vi "CRYGraph Picture Window.vi"() -> ()   [LabVIEW 2013]
uses:
  Control/CRYPicture Property.ctl
  Control/CRYFlag Cluster.ctl
  SubVI/CRYData View Global.vi
  SubVI/CRYMain Sub Window Global.vi
  CRYCurveLibrary/Global/CRYCurve Library Global.vi
panel:
  in  "LoadFinish":bool
  out "Event Name":string
  in  "OpenProperty":bool
  out "PropertyTab":string
  out "Test":string
  in  "Cursor":string[][](table)
  out "Cursor Ref":refnum<vi>
  out "Queue Name":string
  in  "StateOut":bool
  in  "CursorShow":bool
  out "Picture Property":T1
  in  "Draw":bool
  out "Graph Ref":refnum<vi>
  out "Graph Number":i32
  in  "LegendShow":bool
  in  "stop":bool
  out "Legend Ref":refnum<vi>
  in  "Legend":i32(listbox) caption="Multicolumn Listbox"
  in  "GraphType":string
  out "Title Name":string
  out "GPicture":picture
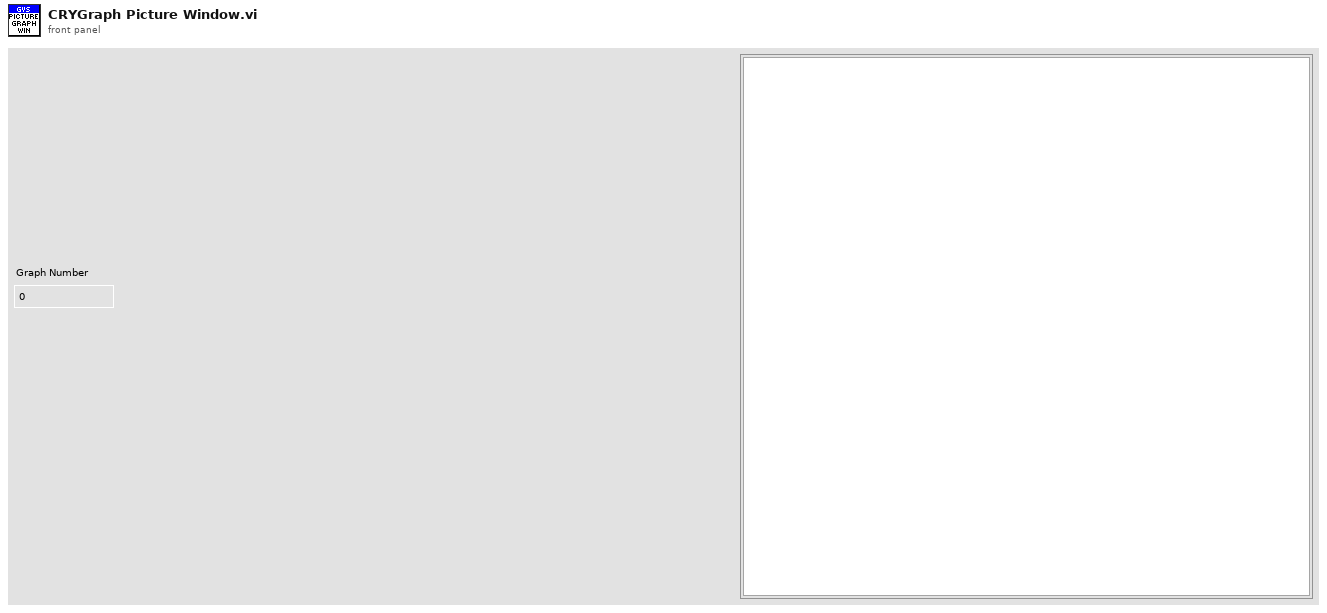
[diagram p1: front panel]
types:
  T1 = typedef "CRYPicture Property.ctl" = cluster{"Image Path":string, "Show vertical scroll bar":bool, "Show horizontal scroll bar":bool}
  T2 = typedef "CRYGraph Event.ctl" = cluster{"EvenName":string, "TitleName":string, "GraphName":string, "GraphType":string, "Data":variant, "Queue Name":string, "DataView Number":i32}
  T3 = typedef "CRYFlag Cluster.ctl" = cluster{"LegendShow":bool, "CellClick":bool, "Total Number":bool, "ScaleFitX":bool, "ScaleFitY":bool, "MapModeX":u8, "MapModeY":u8, "CursorShow":bool, "MagnitudeShow":bool, "PreviewShow":bool, "CursorEnabled":bool, "IntensityShow":bool, "PaletteShow":bool, "PhaseShow":bool, "XYShow":bool, "FrequencyShow":bool, "LegendVScrollShow":bool, "FrequencyVScrollShow":bool}
  T4 = enum16{"Left Button", "Center Button", "Right Button", "Window Close"}
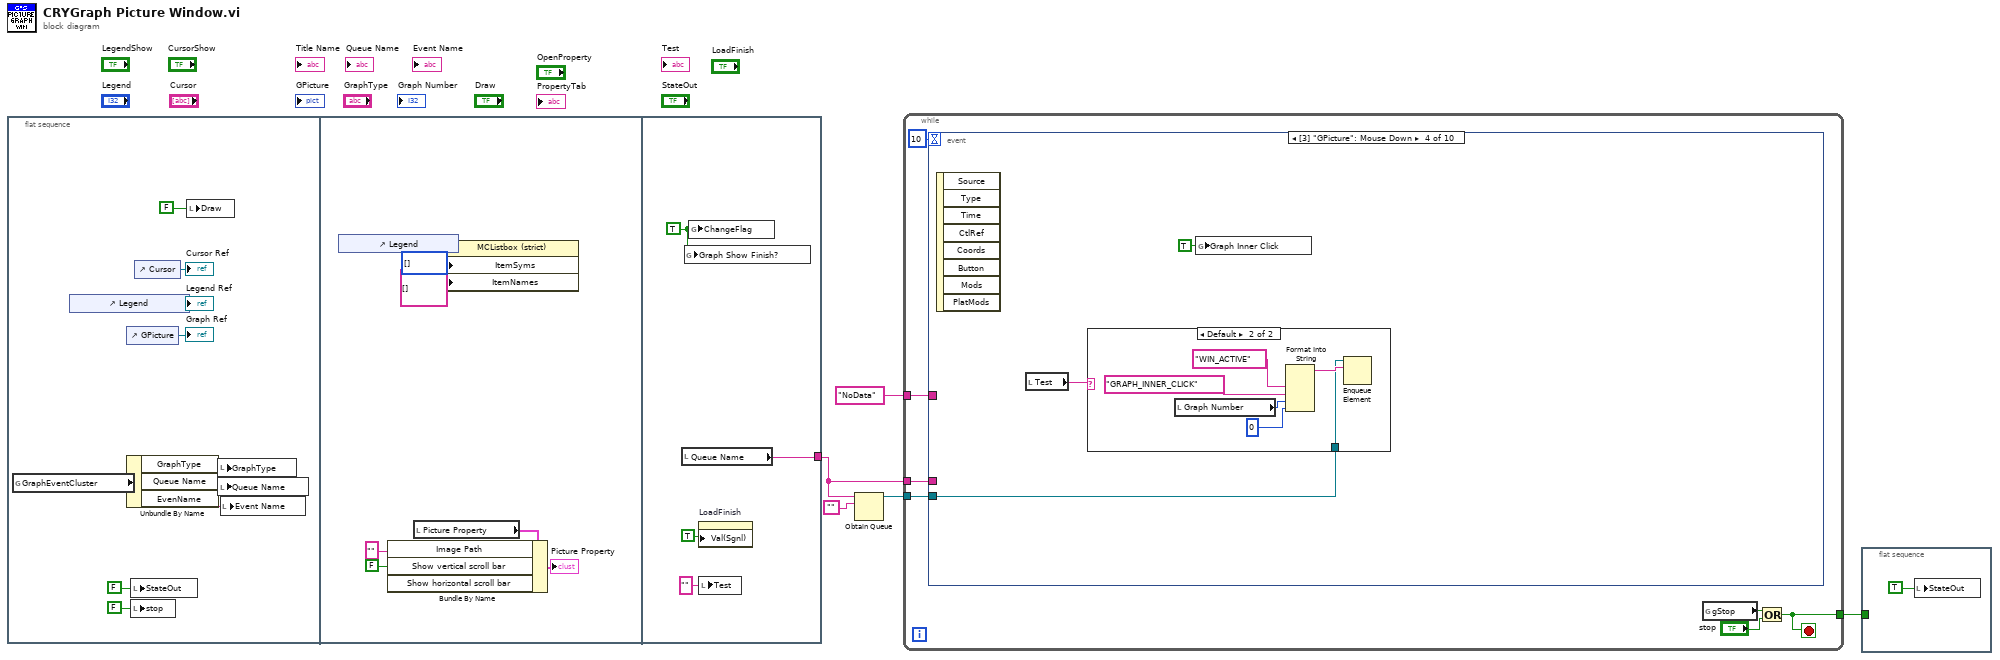
[diagram p0: block diagram]
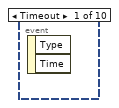
[diagram p2: hidden frame]
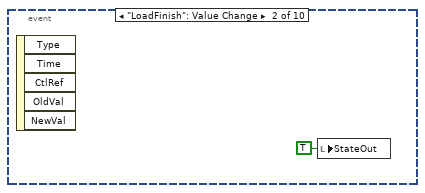
[diagram p3: hidden frame]
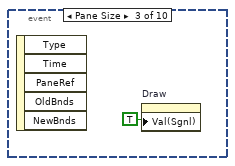
[diagram p4: hidden frame]
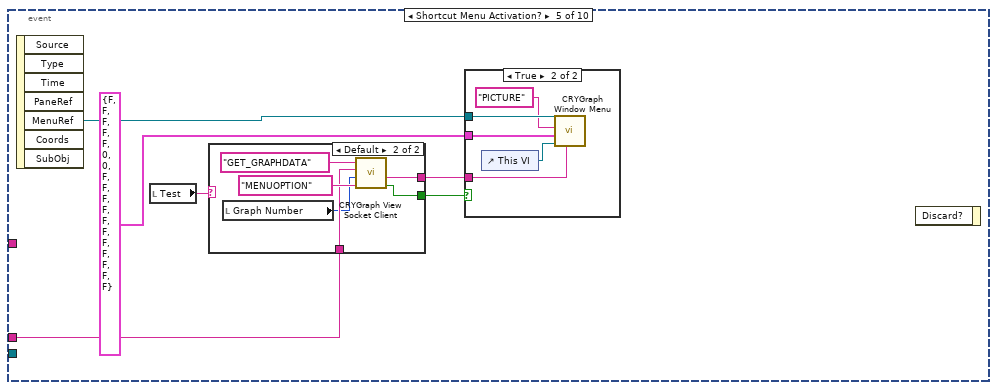
[diagram p6: hidden frame]
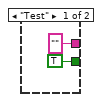
[diagram p7: hidden frame]
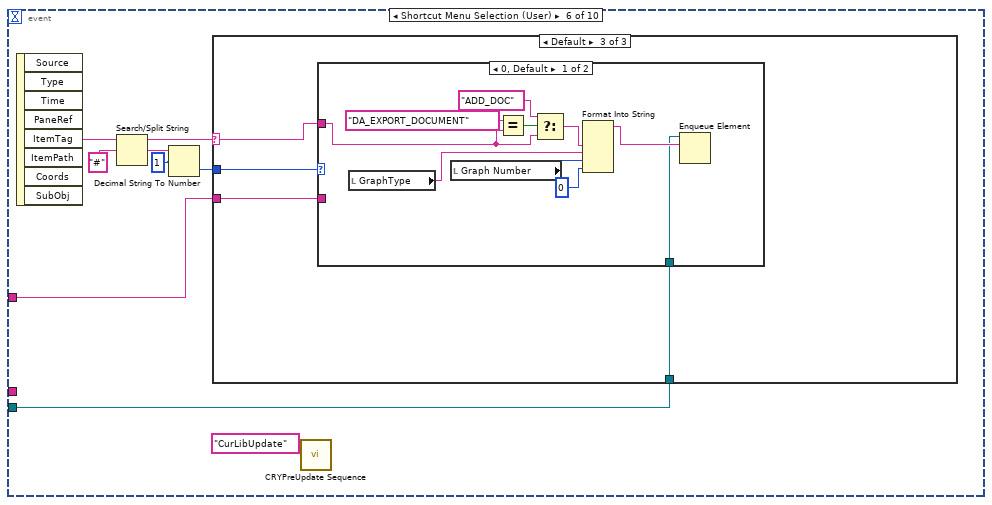
[diagram p9: hidden frame]
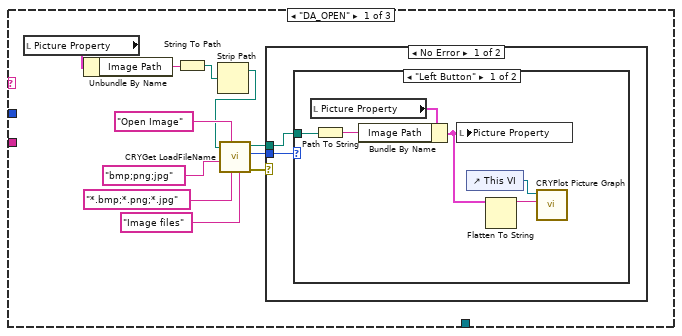
[diagram p10: hidden frame]
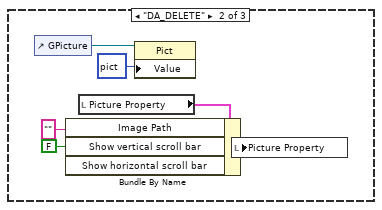
[diagram p13: hidden frame]
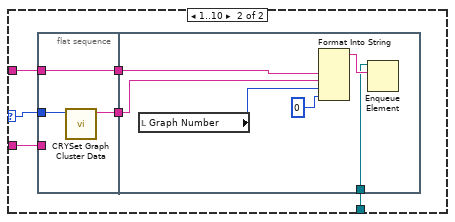
[diagram p14: hidden frame]
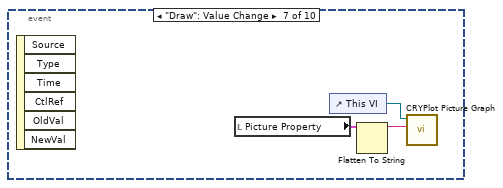
[diagram p15: hidden frame]
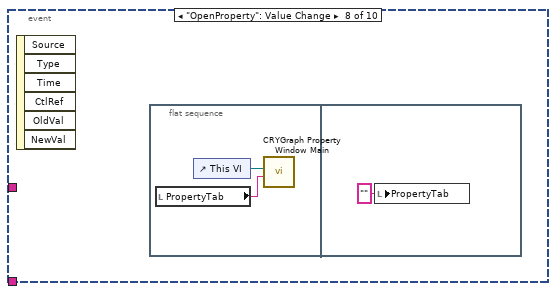
[diagram p16: hidden frame]
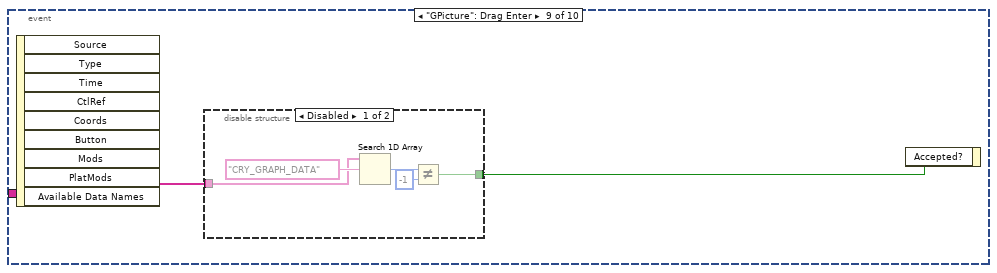
[diagram p17: hidden frame]
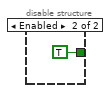
[diagram p18: hidden frame]
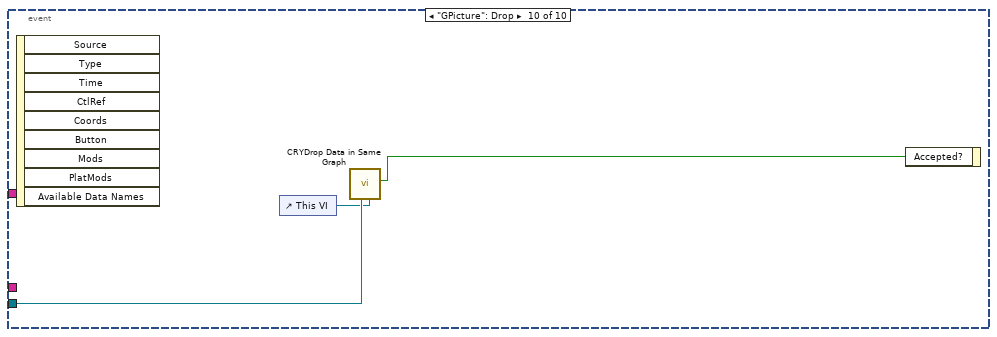
[diagram p19: hidden frame]
diagram:
  n1 = flat-sequence {
    tunnel: [w24] -> w1
    frame #0 {
      n2 = global read "CRYData View Global.vi" "GraphEventCluster"() -> (w8:T2)
      n3 = control-ref of="Legend"() -> (→"Legend Ref":refnum<vi>)
      n4 = control-ref of="GPicture"() -> (→"Graph Ref":refnum<vi>)
      n5 = Unbundle By Name(w8) -> ("GraphType"=w7:string, "Queue Name"=w9:string, "EvenName"=w6:string)
      n6 = local write "StateOut"(FALSE ("StateOut")) -> ()
      n7 = local write "stop"(FALSE ("stop")) -> ()
      n8 = control-ref of="Cursor"() -> (→"Cursor Ref":refnum<vi>)
      n9 = local write "Draw"(FALSE ("Draw")) -> ()
      n10 = local write "GraphType"(w7) -> ()
      n11 = local write "Queue Name"(w9) -> ()
      n12 = local write "Event Name"(w6) -> ()
    }
    frame #1 {
      w22 = FALSE ("Resize Window to Picture")
      n13 = control-ref of="Legend"() -> (w16:refnum<vi>)
      n14 = local read "Picture Property"() -> (w19:T1)
      n15 = Bundle By Name(cluster=w19, "Image Path"="", "Show vertical scroll bar"=w22, "Show horizontal scroll bar"=w22) -> (→"Picture Property":T1)
      n16 = property on="Property Node" class="MCListbox (strict)"(reference=w16, "ItemSyms"=i32[] [] ("Item Symbols"), "ItemNames"=string[][] [] ("Item Names")) -> ()  [unwired: 1 in, 2 out]
    }
    frame #2 {
      w26 = TRUE ("ChangeFlag")
      n17 = local read "Queue Name"() -> (w24:string)
      n18 = global write "CRYData View Global.vi" "Graph Show Finish?"(w26) -> ()
      n19 = global write "CRYData View Global.vi" "ChangeFlag"(w26) -> ()
      n20 = property on="LoadFinish" class="Bool (strict)"("Val(Sgnl)"=TRUE ("Value (Signaling)")) -> ()  [unwired: 2 in, 2 out]
      n21 = local write "Test"("" ("Test")) -> ()
    }
  }
  n22 = Obtain Queue(name (unnamed)=w1, element data type="") -> (queue out=w4:refnum<queue>)  [unwired: 3 in, 2 out]
  n23 = while {
    tunnel: w4 -> [w33]
    tunnel: "NoData" ("input 2") -> [w30]
    tunnel: w1 -> [w28]
    tunnel: [w27] -> w2
    stop <- w27 stop-if-true
    n24 = event shown="[3] \"GPicture\": Mouse Down" {
      selector: _ -> [_ _ _ _ _ _ _ _ _ _]
      dyn-events: _ -> [_ _ _ _ _ _ _ _ _ _]
      timeout: 10 -> [_ _ _ _ _ _ _ _ _ _]
      tunnel: w33 -> [_ _ _ w38 _ w67 _ _ _ w143]
      tunnel: w30 -> [_ _ _ _ _ w66 _ _ _ _]
      tunnel: w28 -> [_ _ _ _ w48 _ _ _ _ _]
      event Timeout {
        n25 = event-data() -> ()  [unwired: 3 out]
      }
      event "LoadFinish": Value Change {
        n26 = event-data() -> ()  [unwired: 6 out]
        n27 = local write "StateOut"(TRUE ("StateOut")) -> ()
      }
      event Pane Size {
        n28 = event-data() -> ()  [unwired: 6 out]
        n29 = property on="Draw" class="Bool (strict)"("Val(Sgnl)"=TRUE ("Value (Signaling)")) -> ()  [unwired: 2 in, 2 out]
      }
      event "GPicture": Mouse Down {
        n30 = event-data() -> ()  [unwired: 9 out]
        n31 = local read "Test"() -> (w37:string)
        n32 = case shown="Default" w37 {
          tunnel: w38 -> [_ w40]
          frame "Test" {
          }
          frame Default {
            n33 = local read "Graph Number"() -> (w44:i32)
            n34 = Format Into String("WIN_ACTIVE" ("input 1"), "GRAPH_INNER_CLICK" ("input 1"), w44, 0 ("input 3")) -> (resulting string=w42:string)  [unwired: 3 in, 1 out]
            n35 = Enqueue Element(queue=w40, element=w42) -> ()  [unwired: 1 in, 4 out]
          }
        }
        n36 = global write "CRYCurve Library Global.vi" "Graph Inner Click"(TRUE ("Graph Inner Click")) -> ()
      }
      event Shortcut Menu Activation? {
        n37 = event-data() -> ("MenuRef"=w47:refnum<k9>)  [unwired: 7 out]
        n38 = local read "Test"() -> (w45:string)
        n39 = case shown="Default" w45 {
          tunnel: ["" ("sData Out") w56] -> w50
          tunnel: [TRUE ("bResult Out") w55] -> w49
          tunnel: w48 -> [_ w54]
          frame "Test" {
          }
          frame Default {
            n40 = local read "Graph Number"() -> (w53:i32)
            n41 = call "CRYGraph View Socket Client.vi"("sOption"="MENUOPTION", "nData"=w53, "sData"=w54, "sAction"="GET_GRAPHDATA") -> ("bResult Out"=w55:bool, "sData Out"=w56:string)  [unwired: 4 in, 2 out]
          }
        }
        n42 = case shown="True" w49 {
          tunnel: w47 -> [_ w63]
          tunnel: T3 {"LegendShow"=FALSE, "CellClick"=FALSE, "Total Number"=FALSE, "ScaleFitX"=FALSE, "ScaleFitY"=FALSE, "MapModeX"=0, "MapModeY"=0, "CursorShow"=FALSE, "MagnitudeShow"=FALSE, "PreviewShow"=FALSE, "CursorEnabled"=FALSE, "IntensityShow"=FALSE, "PaletteShow"=FALSE, "PhaseShow"=FALSE, "XYShow"=FALSE, "FrequencyShow"=FALSE, "LegendVScrollShow"=FALSE, "FrequencyVScrollShow"=FALSE} ("Flag Cluster") -> [_ w61]
          tunnel: w50 -> [_ w60]
          frame False {
          }
          frame True {
            n43 = control-ref of="This VI"() -> (w59:refnum<vi>)
            n44 = call "CRYGraph Window Menu.vi"("MenuOption"=w60, "pGraph VI"=w59, "Flag Cluster"=w61, "Type"="PICTURE", "Runtime Menu Ref In"=w63) -> ()  [unwired: 7 out]
          }
        }
        n45 = event-data() -> ()  [unwired: 1 in, 2 out]
      }
      event Shortcut Menu Selection (User) {
        n46 = event-data() -> ("ItemTag"=w68:string)  [unwired: 8 out]
        n47 = Search/Split String(string=w68, search string/char (-)="#") -> (substring before match=w64:string, match + rest of string=w70:string)  [unwired: 2 out]
        n48 = Decimal String To Number(string=w70, offset=1) -> (number=w72:i32)  [unwired: 2 out]
        n49 = case shown="Default" w64 {
          selector: w64 -> [_ _ w98]
          tunnel: w72 -> [_ _ w101]
          tunnel: w67 -> [_ _ w100]
          tunnel: w66 -> [_ _ w99]
          frame "DA_OPEN" {
            n50 = local read "Picture Property"() -> (w76:T1)
            n51 = Unbundle By Name(w76) -> ("Image Path"=w75:string)
            n52 = String To Path(string=w75) -> (path=w74:path)
            n53 = Strip Path(path=w74) -> (stripped path=w73:path)  [unwired: 1 out]
            n54 = call "CRYGet LoadFileName.vi"("pattern label"="Image files", "pattern (all files)"="*.bmp;*.png;*.jpg", "TitleName"="Open Image" ("Prompt"), "Category Name"="bmp;png;jpg" ("pattern (all files)"), "Start path"=w73) -> ("error out"=w81:errorcluster, "Which Button?"=w77:T4, "Path"=w80:path)  [unwired: 3 in, 1 out]
            n55 = case shown="No Error" w81 {
              tunnel: w77 -> [w85 _]
              tunnel: w80 -> [w84 _]
              frame No Error {
                n56 = case shown="\"Left Button\"" w85 {
                  tunnel: w84 -> [w91 _]
                  frame "Left Button" {
                    n57 = local read "Picture Property"() -> (w90:T1)
                    n58 = Path To String(path=w91) -> (string=w89:string)
                    n59 = Bundle By Name(cluster=w90, "Image Path"=w89) -> (w88:T1)
                    n60 = local write "Picture Property"(w88) -> ()
                    n61 = control-ref of="This VI"() -> (w86:refnum<vi>)
                    n62 = Flatten To String(anything=w88) -> (data string=w87:string)  [unwired: 3 in, 2 out]
                    n63 = call "CRYPlot Picture Graph.vi"("Flattened Property"=w87, "pGraph VI In"=w86) -> ()  [unwired: 10 in]
                  }
                  frame "Center Button", Default {
                  }
                }
              }
              frame Error {
              }
            }
          }
          frame "DA_DELETE" {
            w95 = FALSE ("Resize Window to Picture")
            n64 = control-ref of="GPicture"() -> (w92:refnum<vi>)
            n65 = local read "Picture Property"() -> (w97:T1)
            n66 = Bundle By Name(cluster=w97, "Image Path"="", "Show vertical scroll bar"=w95, "Show horizontal scroll bar"=w95) -> (w94:T1)
            n67 = property class="Pict"(reference=w92, "Value"=picture data[5B]) -> ()  [unwired: 1 in, 2 out]
            n68 = local write "Picture Property"(w94) -> ()
          }
          frame Default {
            n69 = case shown="0, Default" w101 {
              selector: w101 -> [_ w114]
              tunnel: w98 -> [w104 w117]
              tunnel: w100 -> [w109 w116]
              tunnel: w99 -> [_ w113]
              frame 0, Default {
                n70 = local read "GraphType"() -> (w102:string)
                n71 = local read "Graph Number"() -> (w108:i32)
                n72 = Equal?(x="DA_EXPORT_DOCUMENT" ("y"), y=w104) -> (x = y?=w107:bool)
                n73 = Select(t="ADD_DOC", s=w107, f=w104) -> (s? t:f=w103:string)
                n74 = Format Into String(w103, w102, w108, 0 ("input 3")) -> (resulting string=w110:string)  [unwired: 3 in, 1 out]
                n75 = Enqueue Element(queue=w109, element=w110) -> ()  [unwired: 1 in, 4 out]
              }
              frame 1..10 {
                n76 = flat-sequence {
                  tunnel: w117 -> [w120]
                  tunnel: [w120] -> w115
                  tunnel: w114 -> [w119]
                  tunnel: w113 -> [_]
                  tunnel: [w118] -> w112
                  tunnel: w116 -> [w124]
                  tunnel: w115 -> [w123]
                  tunnel: w112 -> [w122]
                  frame #0 {
                    n77 = call "CRYSet Graph Cluster Data.vi"("Graph Number"=w119) -> ("DataType"=w118:string)  [unwired: 2 in, 8 out]
                  }
                  frame #1 {
                    n78 = local read "Graph Number"() -> (w121:i32)
                    n79 = Format Into String(w123, w122, w121, 0 ("input 3")) -> (resulting string=w126:string)  [unwired: 3 in, 1 out]
                    n80 = Enqueue Element(queue=w124, element=w126) -> ()  [unwired: 1 in, 4 out]
                  }
                }
              }
            }
          }
        }
        n81 = call "CRYPreUpdate Sequence.vi"("EventName"="CurLibUpdate") -> ()  [unwired: 15 in]
      }
      event "Draw": Value Change {
        n82 = event-data() -> ()  [unwired: 7 out]
        n83 = local read "Picture Property"() -> (w129:T1)
        n84 = control-ref of="This VI"() -> (w127:refnum<vi>)
        n85 = Flatten To String(anything=w129) -> (data string=w128:string)  [unwired: 3 in, 2 out]
        n86 = call "CRYPlot Picture Graph.vi"("Flattened Property"=w128, "pGraph VI In"=w127) -> ()  [unwired: 10 in]
      }
      event "OpenProperty": Value Change {
        n87 = event-data() -> ()  [unwired: 7 out]
        n88 = flat-sequence {
          frame #0 {
            n89 = local read "PropertyTab"() -> (w130:string)
            n90 = control-ref of="This VI"() -> (w131:refnum<vi>)
            n91 = call "CRYGraph Property Window Main.vi"("TabName"=w130, "pGraph VI In"=w131) -> ()  [unwired: 1 in, 9 out]
          }
          frame #1 {
            n92 = local write "PropertyTab"("" ("PropertyTab")) -> ()
          }
        }
      }
      event "GPicture": Drag Enter {
        n93 = event-data() -> ("Available Data Names"=w134:string[])  [unwired: 9 out]
        n94 = disable-structure shown="Disabled" {
          disable-tunnel: w134 -> [w136 _]
          disable-tunnel: [w135 TRUE] -> w133
          frame Disabled {
            n95 = Search 1D Array(1D array=w136, element="CRY_GRAPH_DATA") -> (index of element=w137:i32)  [unwired: 1 out]
            n96 = Not Equal?(x=w137, y=-1) -> (x != y?=w135:bool)
          }
          frame Enabled {
          }
        }
        n97 = event-data("Accepted?"=w133) -> ()  [unwired: 1 in, 1 out]
      }
      event "GPicture": Drop {
        n98 = event-data() -> ()  [unwired: 10 out]
        n99 = control-ref of="This VI"() -> (w141:refnum<vi>)
        n100 = call "CRYDrop Data in Same Graph.vi"("pGraph VI"=w141, "Queue"=w143) -> ("Accepted?"=w142:bool)  [unwired: 5 in, 4 out]
        n101 = event-data("Accepted?"=w142) -> ()  [unwired: 1 in, 1 out]
      }
    }
    n102 = global read "CRYMain Sub Window Global.vi" "gStop"() -> (w32:bool)
    n103 = Or(x=w32, y="stop") -> (x .or. y?=w27:bool)
  }
  n104 = flat-sequence {
    tunnel: w2 -> [_]
    frame #0 {
      n105 = local write "StateOut"(TRUE ("StateOut")) -> ()
    }
  }
